vi "sched-check.vi"(8 "error in":errorcluster, 9 "stepElement in":variant, 10 "clk":dbl) -> (0 "error out":errorcluster, 1 "stepElement out":variant, 2 "resulting string":string, 4 "Next State":cluster{"CMD":T3, "data":variant})   [LabVIEW 2024]
uses:
  controls/typeCmdPostStepFunc.ctl
  controls/sched-cluster.ctl
  controls/UiScheduleTimestamp.ctl
  controls/typeStepVarients.ctl
  Polymorphics/variantCtrlString.vi
  proc.util.validateParamExist.vi
  <vilib>/Utility/error.llb/Clear Errors.vi
  util.error.create.vi
panel:
  out "stop":timestamp format="%<%X\n%x>T"
  out "start":timestamp format="%<%X\n%x>T"
  out "time stamp":timestamp format="%<%X\n%x>T"
  out "Is Found":bool
  in  "Schedular":T1 {"sched-pairs"."start" format="%<%H:%M %d/%m>T"; "sched-pairs"."stop" format="%<%H:%M %d/%m>T"}
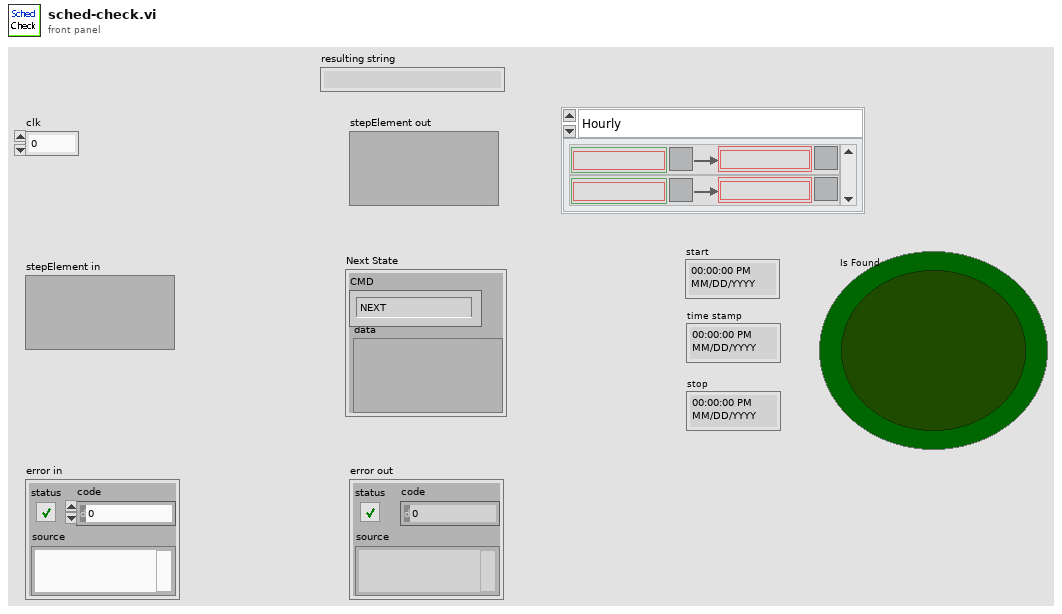
[diagram p1: front panel]
types:
  T1 = typedef "sched-cluster.ctl" = cluster{"sched-mode":enum16{"Hourly", "Daily", "Weekly", "Date"}, "sched-pairs":cluster{"start":T2, "stop":T2}[]}
  T2 = typedef "UiScheduleTimestamp.ctl" = timestamp
  T3 = typedef "typeCmdPostStepFunc.ctl" = enum16{"NEXT", "PREV", "JUMP", "STAY", "COMPLETE", "ENGCALL.PROC.START", "ENGCALL.PROC.STOP", "ENGCALL.PROC.COMPLETION-CHECK", "ENGCALL.PROC.INIT", "ERROR"}
  T4 = typedef "typeStepVarients.ctl" = enum16{"stepNameID", "stepFunction", "stepReport", "stepSetpoint", "stepPointer", "stepProcPointer", "stepIoPointer", "stepIoValue", "stepFilePointer", "stepMessage", "stepTimeString", "stepNumReg", "stepStrReg", "stepSeconds", "stepUnitDoseParams", "stepUnitIndex"}
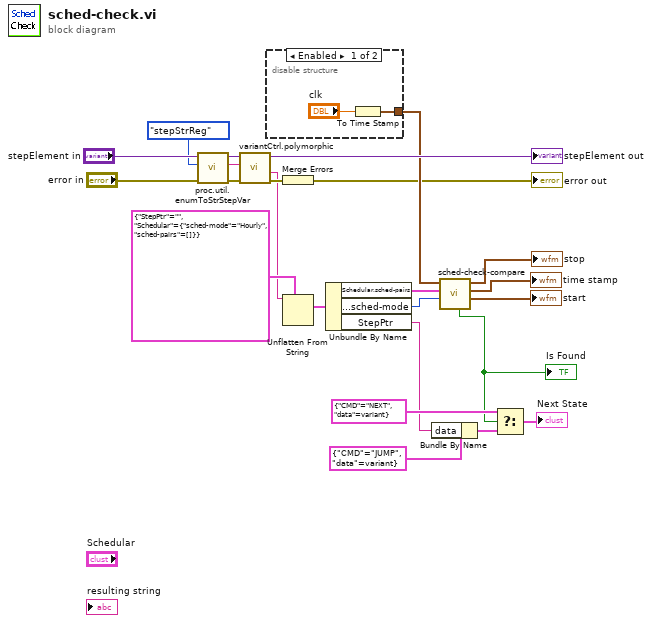
[diagram p0: block diagram]
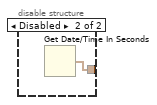
[diagram p2: hidden frame]
diagram:
  n1 = call "proc.util.enumToStrStepVar.vi"("Step var"=typeStepVarients."stepStrReg") -> ("String"=w16:string)  [unwired: 10 in]
  n2 = call-poly "variantCtrl.polymorphic.vi"("error in"="error in", "name in"=w16, "Step in"="stepElement in") -> ("error out"=w11:errorcluster, "String Value"=w7:string, "Step out"=→"stepElement out":variant)  [unwired: 5 in, 1 out]
  n3 = disable-structure shown="Enabled" {
    disable-tunnel: [w23 w25] -> w2
    frame Enabled {
      n4 = To Time Stamp(1:"clk") -> (0:w23:timestamp)
    }
    frame Disabled {
      n5 = Get Date/Time In Seconds() -> (seconds since 1Jan1904=w25:timestamp)
    }
  }
  n6 = Merge Errors(w11) -> (→"error out":errorcluster)
  n7 = Unflatten From String(type=cluster{"StepPtr":string, "Schedular":T1} {"StepPtr"="", "Schedular"={"sched-mode"=enum."Hourly", "sched-pairs"=[]}} ("output cluster"), binary string=w7) -> (value=w8:cluster{"StepPtr":string, "Schedular":T1})  [unwired: 3 in, 2 out]
  n8 = Unbundle By Name(w8) -> ("Schedular.sched-pairs"=w21:cluster{"start":T2, "stop":T2}[], "Schedular.sched-mode"=w22:enum16{"Hourly", "Daily", "Weekly", "Date"}, "StepPtr"=w6:string)
  n9 = Bundle By Name(cluster=cluster{"CMD":T3, "data":variant} {"CMD"=enum."JUMP", "data"=variant} ("JUMP"), "data"=w6) -> (w14:cluster{"CMD":T3, "data":variant})
  n10 = call "sched-check-compare.vi"("sched-mode"=w22, "sched-pairs"=w21, "time stamp"=w2) -> ("Start"=→"start":timestamp, "Time"=→"time stamp":timestamp, "Stop"=→"stop":timestamp, "Found?"=w10:bool)  [unwired: 5 in]
  "Is Found" <- w10
  n11 = Select(t=cluster{"CMD":T3, "data":variant} {"CMD"=enum."NEXT", "data"=variant} ("NEXT"), s=w10, f=w14) -> (s? t:f=→"Next State":cluster{"CMD":T3, "data":variant})
